vi "LoginForm.vi"(2 "DBSet":T1) -> (0 "登录成功":bool, 1 "用户名":string, 3 "loginMode":bool, 4 "厂区":string)   [LabVIEW 2011]
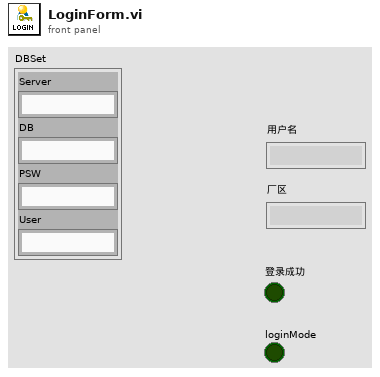
[diagram p1: front panel]
types:
  T1 = cluster{"Server":string, "DB":string, "PSW":string, "User":string}
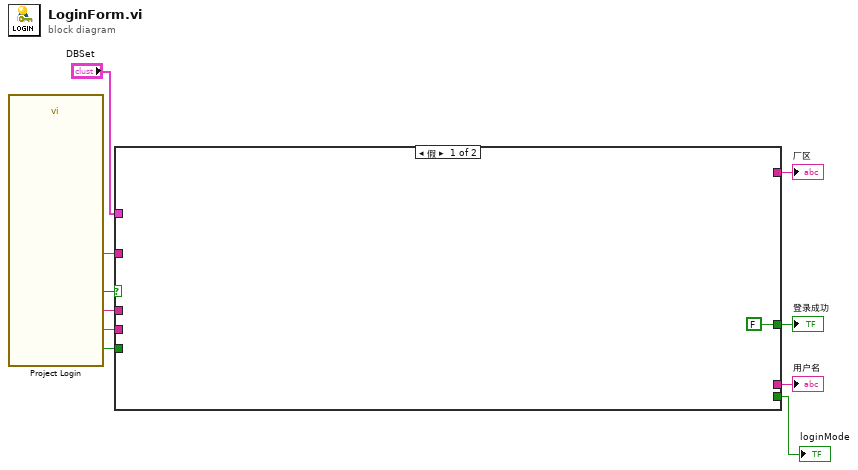
[diagram p0: block diagram]
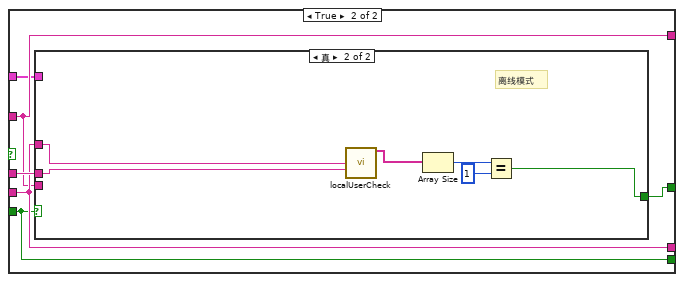
[diagram p2: hidden frame]
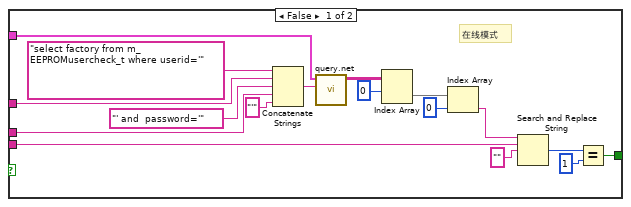
[diagram p3: hidden frame]
diagram:
  n1 = call "Project Login.vi"() -> ("厂区"=w7:string, "mode"=w2:bool, "密码"=w8:string, "用户名"=w9:string, "登录"=w10:bool)  [unwired: 14 in, 1 out]
  n2 = case shown="假" w10 {
    tunnel: w9 -> [_ w16]
    tunnel: w8 -> [_ w17]
    tunnel: w7 -> [_ w15]
    tunnel: [_ w16] -> w6
    tunnel: [_ w15] -> w4
    tunnel: [FALSE w13] -> w5
    tunnel: "DBSet" -> [_ w14]
    tunnel: w2 -> [_ w12]
    tunnel: [_ w12] -> w1
    frame False {
    }
    frame True {
      n3 = case shown="真" w12 {
        tunnel: w17 -> [w32 w39]
        tunnel: w16 -> [w23 w40]
        tunnel: w15 -> [w22 _]
        tunnel: w14 -> [w19 _]
        tunnel: [w18 w35] -> w13
        frame False {
          # "在线模式"
          n4 = Concatenate Strings("select factory from m_EEPROMusercheck_t where userid='", w23, "' and  password='", w32, "'" ("字符串")) -> (w21:string)
          n5 = call "query.net.vi"("Sql"=w21, "DBSet"=w19) -> ("result"=w20:string[][])  [unwired: 8 in, 1 out]
          n6 = Index Array(array=w20, index (row)=0 ("索引 (行)")) -> (element=w30:string[])  [unwired: 1 in]
          n7 = Index Array(array=w30, index=0 ("索引")) -> (element=w28:string)
          n8 = Search and Replace String(input string=w28, search string=w22, replace string="" ("替换字符串(\"\")")) -> (number of replacements=w26:i32)  [unwired: 5 in, 3 out]
          n9 = Equal?(x=w26, y=1) -> (x = y?=w18:bool)
        }
        frame True {
          # "离线模式"
          n10 = call "localUserCheck.vi"("name"=w40, "psw"=w39) -> ("userList"=w38:string[])  [unwired: 12 in, 1 out]
          n11 = Array Size(array=w38) -> (size(s)=w37:i32)
          n12 = Equal?(x=w37, y=1) -> (x = y?=w35:bool)
        }
      }
    }
  }
  "用户名" <- w6
  "登录成功" <- w5
  "厂区" <- w4
  "loginMode" <- w1
